vi "Autoscale Image.vi"(8 "error in (no error)":errorcluster, 10 "Autoscale":bool, 11 "Refnum in":T1) -> (0 "error out":errorcluster, 3 "Refnum out":T1)   [LabVIEW 2013]
uses:
  <vilib>/vision/Image Controls.llb/IMAQ Image.ctl
  <vilib>/vision/NI_Vision_Development_Module.lvlib
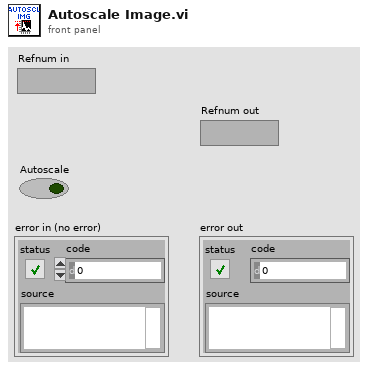
[diagram p1: front panel]
types:
  T1 = typedef "IMAQ Image.ctl" = refnum<image>
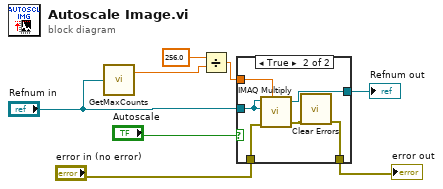
[diagram p0: block diagram]
diagram:
  n1 = call "GetMaxCounts.vi"("New Image"="Refnum in") -> ("Maximal Value"=w1:sgl)  [unwired: 1 out]
  n2 = Divide(x=256.0, y=w1) -> (x/y=w4:dbl)
  n3 = case shown="True" "Autoscale" {
    tunnel: "Refnum in" -> [w10 w13]
    tunnel: w4 -> [_ w16]
    tunnel: [w10 w14] -> w6
    tunnel: "error in (no error)" -> [w9 w12]
    tunnel: [w9 w11] -> w8
    frame False {
    }
    frame True {
      n4 = call "IMAQ Multiply"("Image Src A"=w13, "Constant"=w16, "Image Dst"=w13, "error in (no error)"=w12) -> ("Image Dst Out"=w14:T1, "error out"=w15:errorcluster)  [unwired: 3 in]
      n5 = call <vilib>:"Clear Errors.vi"("error in (no error)"=w15) -> ("error out"=w11:errorcluster)  [unwired: 6 in]
    }
  }
  "error out" <- w8
  "Refnum out" <- w6
